vi "Controller Drive.vi"(0 "input cluster":T2) -> (14 "Strafe":dbl, 15 "Forward/Reverse":dbl, 16 "Turn":dbl, 17 "Picker Upper Up":bool, 18 "Picker Upper Down":bool)   [LabVIEW 2013]
uses:
  <vilib>/Rock Robotics/WPI/Joystick/WPI_JoystickButtonState.ctl
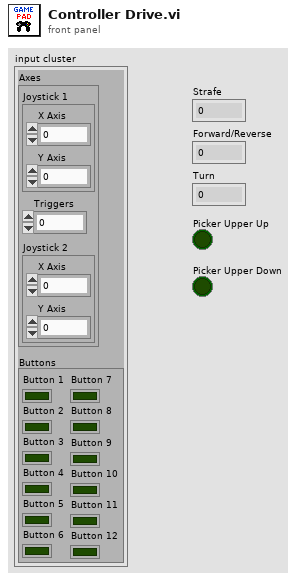
[diagram p1: front panel]
types:
  T1 = typedef "WPI_JoystickButtonState.ctl" = cluster{"Button 1":bool, "Button 2":bool, "Button 3":bool, "Button 4":bool, "Button 5":bool, "Button 6":bool, "Button 7":bool, "Button 8":bool, "Button 9":bool, "Button 10":bool, "Button 11":bool, "Button 12":bool}
  T2 = cluster{"Axes":cluster{"Joystick 1":cluster{"X Axis":dbl, "Y Axis":dbl}, "Triggers":dbl, "Joystick 2":cluster{"X Axis":dbl, "Y Axis":dbl}}, "Buttons":T1}
  T3 = cluster{"Joystick 1":cluster{"X Axis":dbl, "Y Axis":dbl}, "Triggers":dbl, "Joystick 2":cluster{"X Axis":dbl, "Y Axis":dbl}}
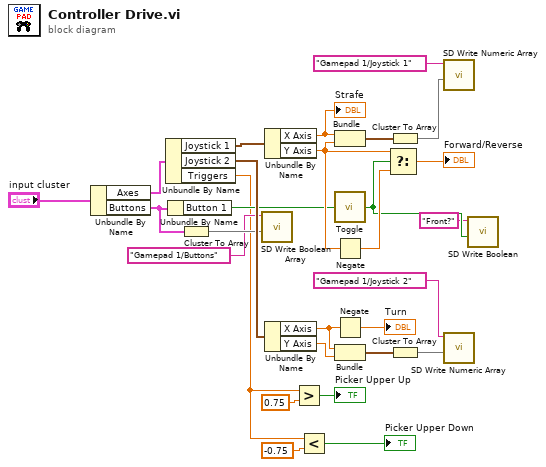
[diagram p0: block diagram]
diagram:
  n1 = Unbundle By Name("input cluster") -> ("Axes"=w28:T3, "Buttons"=w8:T1)
  n2 = Unbundle By Name(w28) -> ("Joystick 1"=w27:cluster{"X Axis":dbl, "Y Axis":dbl}, "Joystick 2"=w18:cluster{"X Axis":dbl, "Y Axis":dbl}, "Triggers"=w3:dbl)
  n3 = Unbundle By Name(w8) -> ("Button 1"=w7:bool)
  n4 = Cluster To Array(cluster=w8) -> (array=w10:bool[])
  n5 = call <vilib>:"SD Write Boolean Array.vi"("Boolean Array"=w10, "Name"="Gamepad 1/Buttons") -> ()  [unwired: 8 in, 2 out]
  n6 = Unbundle By Name(w27) -> ("X Axis"=w26:dbl, "Y Axis"=w15:dbl)
  "Strafe" <- w26
  n7 = Unbundle By Name(w18) -> ("X Axis"=w19:dbl, "Y Axis"=w21:dbl)
  n8 = Greater?(x=w3, y=0.75) -> (0:→"Picker Upper Up":bool)
  n9 = Less?(x=w3, y=-0.75) -> (x < y?=→"Picker Upper Down":bool)
  n10 = Bundle("X Axis"=w26, "Y Axis"=w15) -> (w16:cluster{"X Axis":dbl, "Y Axis":dbl})  [unwired: 1 in]
  n11 = call "Toggle.vi"("Input"=w7) -> ("Latched"=w2:bool)
  n12 = Negate(x=w15) -> (-x=w14:dbl)
  n13 = Negate(x=w19) -> (-x=→"Turn":dbl)
  n14 = Bundle("X Axis"=w19, "Y Axis"=w21) -> (w23:cluster{"X Axis":dbl, "Y Axis":dbl})  [unwired: 1 in]
  n15 = Select(t=w15, s=w2, f=w14) -> (s? t:f=→"Forward/Reverse":dbl)
  n16 = Cluster To Array(cluster=w16) -> (array=w25:dbl[])
  n17 = Cluster To Array(cluster=w23) -> (array=w22:dbl[])
  n18 = call <vilib>:"SD Write Numeric Array.vi"("Numeric Array"=w25, "Name"="Gamepad 1/Joystick 1") -> ()  [unwired: 8 in, 2 out]
  n19 = call <vilib>:"SD Write Numeric Array.vi"("Numeric Array"=w22, "Name"="Gamepad 1/Joystick 2") -> ()  [unwired: 8 in, 2 out]
  n20 = call <vilib>:"SD Write Boolean.vi"("Boolean"=w2, "Name"="Front?") -> ()  [unwired: 8 in, 2 out]
